vi "umbrales.vi"() -> ()   [LabVIEW 2018]
uses:
  Control 1.ctl
panel:
  out "alarma1":bool
  out "alarma2":bool
  out "alarma3":bool
  in  "ntc":dbl
  in  "pt100":dbl
  in  "lm35":dbl
  out "led 3":bool
  out "led 2":bool
  out "led1":bool
  out "sensor ntc":dbl(knob) scale=0.0..100.0
  out "sensor pt100":dbl(knob) scale=0.0..100.0
  out "sensor lm35":dbl(knob) scale=0.0..100.0
  in  "Umbral min 3":dbl
  in  "Umbral max 3":dbl
  in  "Umbral min 2":dbl
  in  "Umbral max 2":dbl
  in  "Umbral min 1":dbl
  in  "Umbral max 1":dbl
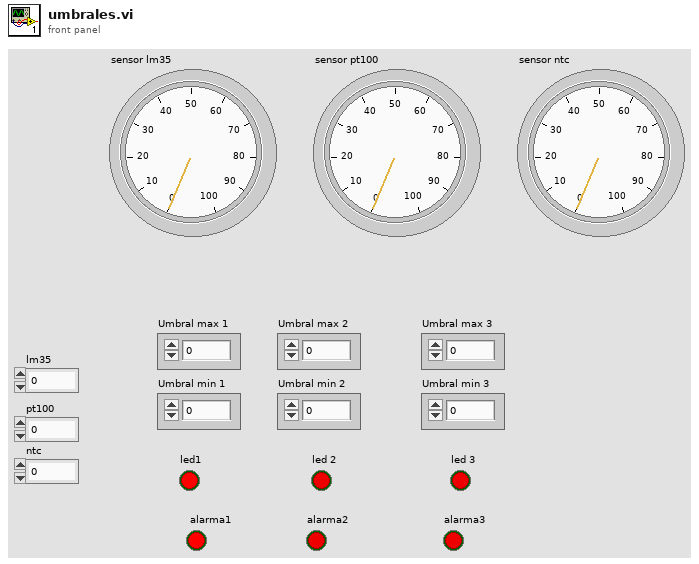
[diagram p1: front panel]
types:
  T1 = typedef "Control 1.ctl" = enum16{"inicio", "alarma1", "alarmal2", "alarmal3"}
  T2 = enum16{"open", "replace", "create", "open or create", "replace or create", "replace or create with confirmation"}
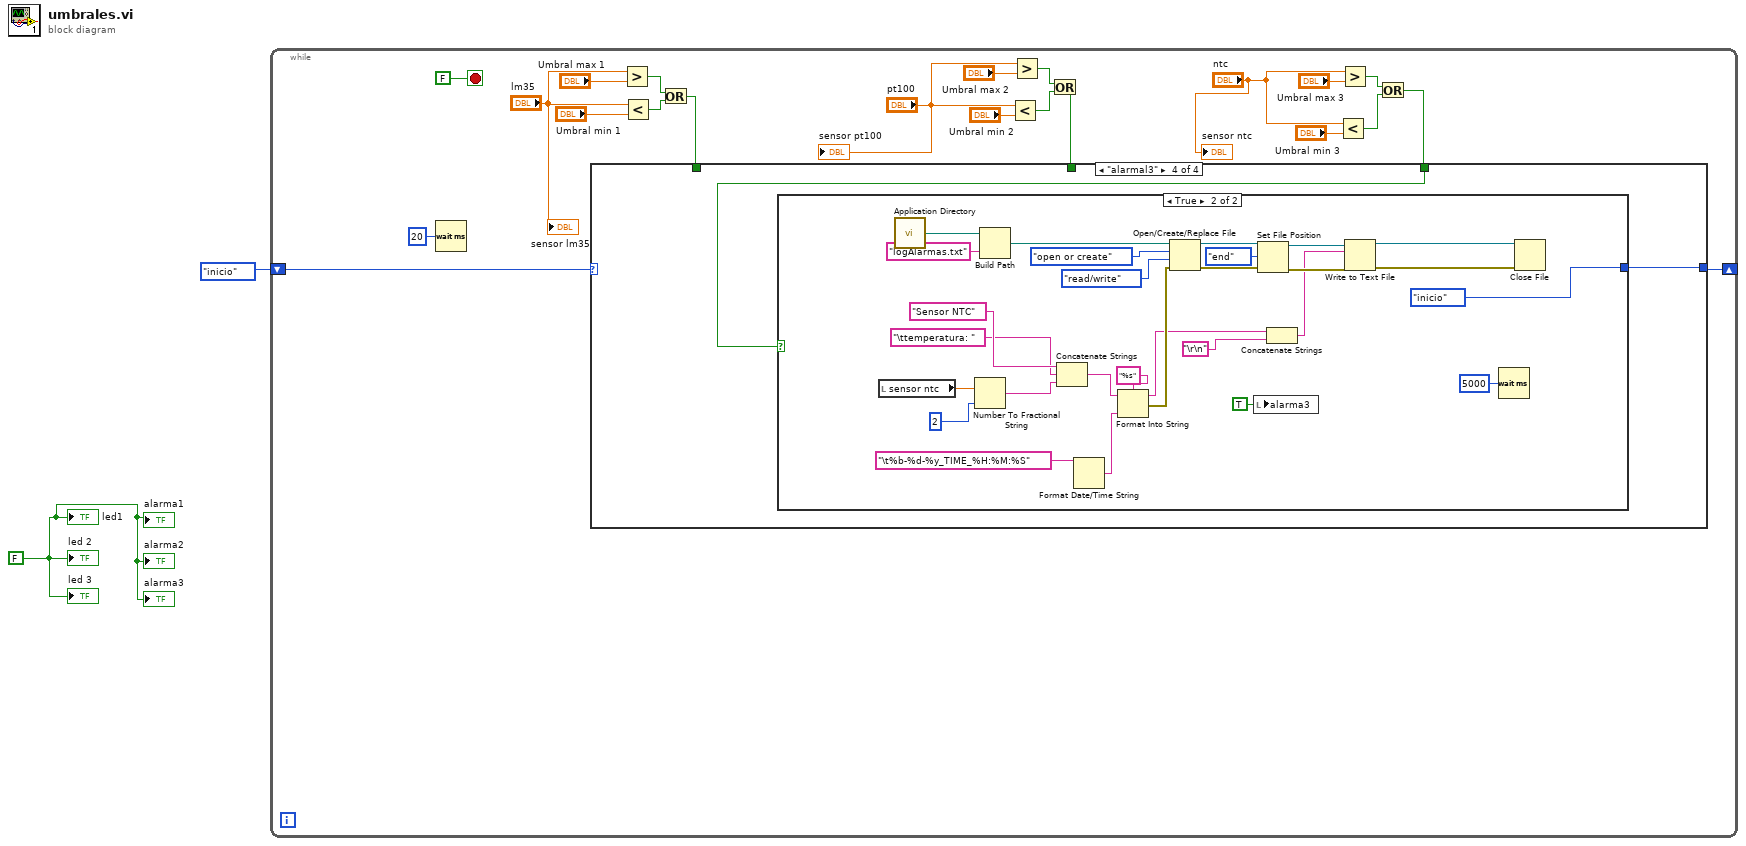
[diagram p0: block diagram]
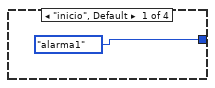
[diagram p2: hidden frame]
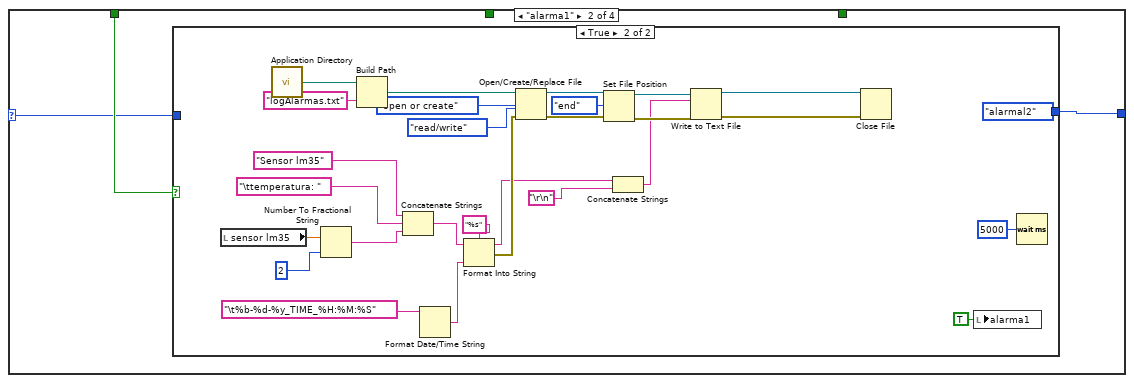
[diagram p3: hidden frame]
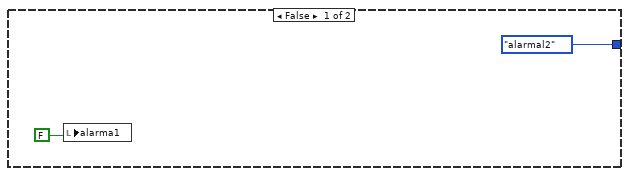
[diagram p4: hidden frame]
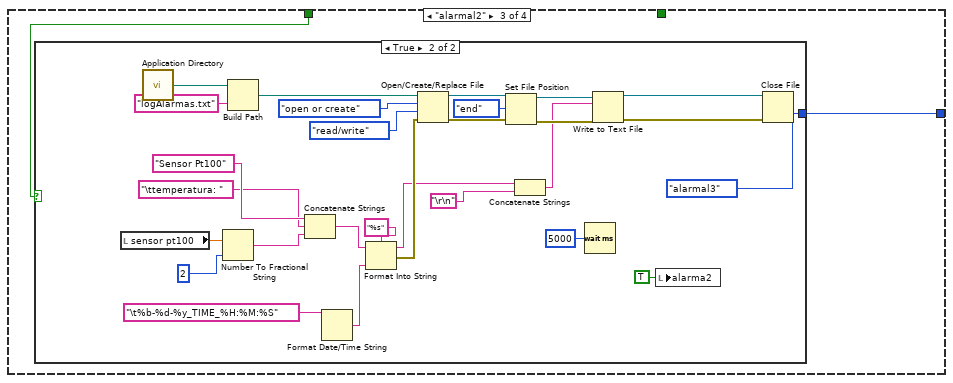
[diagram p5: hidden frame]
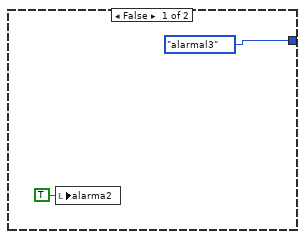
[diagram p6: hidden frame]
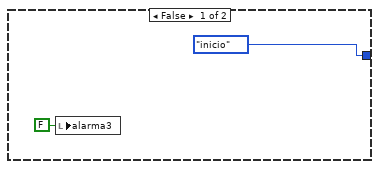
[diagram p7: hidden frame]
diagram:
  w2 = FALSE ("led1")
  n1 = while {
    shift-right: [w17] -> _
    shift-left: Control_1."inicio" -> [w23]
    stop <- FALSE stop-if-true
    n2 = Wait (ms)(milliseconds to wait=u32 20) -> ()  [unwired: 1 out]
    n3 = Greater?(x="lm35", y="Umbral max 1") -> (0:w19:bool)
    n4 = Less?(x="lm35", y="Umbral min 1") -> (x < y?=w18:bool)
    n5 = Or(x=w19, y=w18) -> (x .or. y?=w8:bool)
    n6 = Less?(x="pt100", y="Umbral min 2") -> (x < y?=w14:bool)
    n7 = Greater?(x="pt100", y="Umbral max 2") -> (0:w13:bool)
    n8 = Or(x=w13, y=w14) -> (x .or. y?=w7:bool)
    n9 = Less?(x="ntc", y="Umbral min 3") -> (x < y?=w10:bool)
    n10 = Greater?(x="ntc", y="Umbral max 3") -> (0:w9:bool)
    n11 = Or(x=w9, y=w10) -> (x .or. y?=w6:bool)
    n12 = case shown="\"alarmal3\"" w23 {
      selector: w23 -> [_ w26 _ _]
      tunnel: [Control_1."alarma1" w28 w60 w92] -> w17
      tunnel: w8 -> [_ w27 _ _]
      tunnel: w7 -> [_ _ w59 _]
      tunnel: w6 -> [_ _ _ w91]
      frame "inicio", Default {
      }
      frame "alarma1" {
        n13 = case shown="True" w27 {
          tunnel: [Control_1."alarmal2" Control_1."alarmal2"] -> w28
          tunnel: w26 -> [_ _]
          frame False {
            n14 = local write "alarma1"(FALSE ("led1")) -> ()
          }
          frame True {
            n15 = local read "sensor lm35"() -> (w38:dbl)
            n16 = call <vilib>:"Application Directory.vi"() -> ("Application Directory"=w57:path)
            n17 = Number To Fractional String(number=w38, precision (6)=i16 2) -> (F-format string=w35:string)  [unwired: 2 in]
            n18 = Build Path(base path=w57, name or relative path="logAlarmas.txt") -> (appended path=w56:path)
            n19 = Concatenate Strings("Sensor lm35" ("format string"), "\ttemperatura: " ("format string"), w35) -> (w34:string)
            n20 = Format Date/Time String(time format string (%c)="\t%b-%d-%y_TIME_%H:%M:%S") -> (date/time string=w42:string)  [unwired: 2 in]
            n21 = Format Into String(format string="%s", initial string=w34, w42) -> (resulting string=w40:string, error out=w44:errorcluster)  [unwired: 1 in]
            n22 = Open/Create/Replace File(file path (use dialog)=w56, error in=w44, operation (0:open)=T2."open or create", access (0:read/write)=enum16{"read/write", "read-only", "write-only"}."read/write") -> (refnum out=w52:refnum<file>, error out=w51:errorcluster)  [unwired: 2 in, 1 out]
            n23 = Set File Position(refnum=w52, from (0:start)=enum16{"start", "end", "current"}."end", error in=w51) -> (refnum out=w49:refnum<file>, error out=w48:errorcluster)  [unwired: 1 in]
            n24 = Concatenate Strings(w40, "\r\n") -> (w39:string)
            n25 = Write to Text File(file (use dialog)=w49, text=w39, error in=w48) -> (refnum out=w47:refnum<file>, error out=w46:errorcluster)  [unwired: 1 in, 1 out]
            n26 = Close File(refnum=w47, error in=w46) -> ()  [unwired: 2 out]
            n27 = local write "alarma1"(TRUE ("led1")) -> ()
            n28 = Wait (ms)(milliseconds to wait=u32 5000) -> ()  [unwired: 1 out]
          }
        }
      }
      frame "alarmal2" {
        n29 = case shown="True" w59 {
          tunnel: [Control_1."alarmal3" Control_1."alarmal3"] -> w60
          frame False {
            n30 = local write "alarma2"(TRUE ("led1")) -> ()
          }
          frame True {
            n31 = local read "sensor pt100"() -> (w78:dbl)
            n32 = call <vilib>:"Application Directory.vi"() -> ("Application Directory"=w90:path)
            n33 = Number To Fractional String(number=w78, precision (6)=i16 2) -> (F-format string=w77:string)  [unwired: 2 in]
            n34 = Build Path(base path=w90, name or relative path="logAlarmas.txt") -> (appended path=w89:path)
            n35 = Concatenate Strings("Sensor Pt100" ("format string"), "\ttemperatura: " ("format string"), w77) -> (w76:string)
            n36 = Format Date/Time String(time format string (%c)="\t%b-%d-%y_TIME_%H:%M:%S") -> (date/time string=w81:string)  [unwired: 2 in]
            n37 = Format Into String(format string="%s", initial string=w76, w81) -> (resulting string=w80:string, error out=w82:errorcluster)  [unwired: 1 in]
            n38 = Open/Create/Replace File(file path (use dialog)=w89, error in=w82, operation (0:open)=T2."open or create", access (0:read/write)=enum16{"read/write", "read-only", "write-only"}."read/write") -> (refnum out=w88:refnum<file>, error out=w87:errorcluster)  [unwired: 2 in, 1 out]
            n39 = Set File Position(refnum=w88, from (0:start)=enum16{"start", "end", "current"}."end", error in=w87) -> (refnum out=w86:refnum<file>, error out=w85:errorcluster)  [unwired: 1 in]
            n40 = Concatenate Strings(w80, "\r\n") -> (w79:string)
            n41 = Wait (ms)(milliseconds to wait=u32 5000) -> ()  [unwired: 1 out]
            n42 = Write to Text File(file (use dialog)=w86, text=w79, error in=w85) -> (refnum out=w84:refnum<file>, error out=w83:errorcluster)  [unwired: 1 in, 1 out]
            n43 = local write "alarma2"(TRUE ("led1")) -> ()
            n44 = Close File(refnum=w84, error in=w83) -> ()  [unwired: 2 out]
          }
        }
      }
      frame "alarmal3" {
        n45 = case shown="True" w91 {
          tunnel: [Control_1."inicio" Control_1."inicio"] -> w92
          frame False {
            n46 = local write "alarma3"(FALSE ("led1")) -> ()
          }
          frame True {
            n47 = local read "sensor ntc"() -> (w108:dbl)
            n48 = call <vilib>:"Application Directory.vi"() -> ("Application Directory"=w120:path)
            n49 = Number To Fractional String(number=w108, precision (6)=i16 2) -> (F-format string=w107:string)  [unwired: 2 in]
            n50 = Build Path(base path=w120, name or relative path="logAlarmas.txt") -> (appended path=w119:path)
            n51 = Concatenate Strings("Sensor NTC" ("format string"), "\ttemperatura: " ("format string"), w107) -> (w106:string)
            n52 = Format Date/Time String(time format string (%c)="\t%b-%d-%y_TIME_%H:%M:%S") -> (date/time string=w111:string)  [unwired: 2 in]
            n53 = Format Into String(format string="%s", initial string=w106, w111) -> (resulting string=w110:string, error out=w112:errorcluster)  [unwired: 1 in]
            n54 = Open/Create/Replace File(file path (use dialog)=w119, error in=w112, operation (0:open)=T2."open or create", access (0:read/write)=enum16{"read/write", "read-only", "write-only"}."read/write") -> (refnum out=w118:refnum<file>, error out=w117:errorcluster)  [unwired: 2 in, 1 out]
            n55 = local write "alarma3"(TRUE ("led1")) -> ()
            n56 = Set File Position(refnum=w118, from (0:start)=enum16{"start", "end", "current"}."end", error in=w117) -> (refnum out=w116:refnum<file>, error out=w115:errorcluster)  [unwired: 1 in]
            n57 = Concatenate Strings(w110, "\r\n") -> (w109:string)
            n58 = Write to Text File(file (use dialog)=w116, text=w109, error in=w115) -> (refnum out=w114:refnum<file>, error out=w113:errorcluster)  [unwired: 1 in, 1 out]
            n59 = Wait (ms)(milliseconds to wait=u32 5000) -> ()  [unwired: 1 out]
            n60 = Close File(refnum=w114, error in=w113) -> ()  [unwired: 2 out]
          }
        }
      }
    }
    "sensor pt100" <- "pt100"
    "sensor ntc" <- "ntc"
    "sensor lm35" <- "lm35"
  }
  "led1" <- w2
  "led 2" <- w2
  "led 3" <- w2
  "alarma1" <- w2
  "alarma2" <- w2
  "alarma3" <- w2
